vi "Impulsi START STOP.vi"(11 "Segnale":bool) -> (2 "STOP":bool, 3 "START":bool)   [LabVIEW 2019]
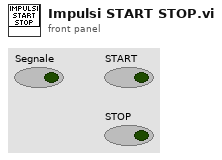
[diagram p1: front panel]
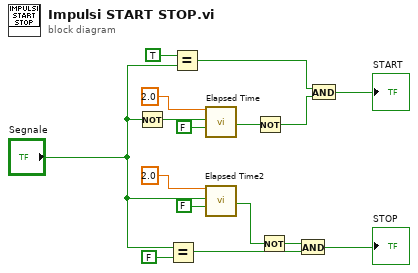
[diagram p0: block diagram]
diagram:
  n1 = Not(x="Segnale") -> (.not. x?=w4:bool)
  n2 = Equal?(x="Segnale", y=FALSE) -> (x = y?=w13:bool)
  n3 = Equal?(x=TRUE, y="Segnale") -> (x = y?=w6:bool)
  n4 = call "Elapsed Time"("Time Target (s)"=2.0, "Reset"=w4, "Auto Reset"=FALSE) -> ("Time has Elapsed"=w7:bool)  [unwired: 9 in, 7 out]
  n5 = call "Elapsed Time2"("Time Target (s)"=2.0, "Reset"="Segnale", "Auto Reset"=FALSE) -> ("Time has Elapsed"=w14:bool)  [unwired: 9 in, 7 out]
  n6 = Not(x=w7) -> (.not. x?=w8:bool)
  n7 = Not(x=w14) -> (.not. x?=w15:bool)
  n8 = And(x=w15, y=w13) -> (x .and. y?=→"STOP":bool)
  n9 = And(x=w6, y=w8) -> (x .and. y?=→"START":bool)
